vi "Create.vi"(7 "Direction":T1, 8 "error in (no error)":errorcluster, 9 "Custom Config Data":u8[](array[numeric]), 10 "Name":string, 11 "CIF_NIChn_FIFO_DAQ in":refnum<class "CIF_NIChn_DAQ_Base.lvclass">) -> (0 "error out":errorcluster, 3 "CIF_NIChn_FIFO_DAQ out":refnum<class "CIF_NIChn_DAQ_Base.lvclass">)   [LabVIEW 2021, in "CIF_NIChn_DAQ_Base.lvclass"]
uses:
  CIF_NIChn_DAQ_Base.lvclass
  D:/dev/Packages/CIF_Channels_Core/src/CIFChannels/CIFChannels.lvclass
  D:/dev/Packages/CIF_Channels_Core/src/CIF_NIChn/NIChn/CIF_NIChn.lvclass
  D:/dev/Packages/CIF_Channels_Core/src/CIF_NIChn/FIFO_U8/CIF_NIChn_Fifo_U8.lvclass
  CIFChannels/Typedef/Direction.ctl
  <vilib>/CIF Foundation/CIF Utilities/Statistics/I64/Stats_I64_CIF_U.lvclass/Stats_I64_CIF_U.ctl
  CIFChannels/Typedef/Disconnect Behavior.ctl
  CIFChannels/CIFChannels.lvclass/CIFChannels.ctl
  Typedef/Datatype Waveform Channel.ctl
  CIFChannels/Typedef/Channel State.ctl
  CIF_NIChn_DAQ_Base.lvclass/CIF_NIChn_DAQ_Base.ctl
  NIChn/CIF_NIChn.lvclass/CIF_NIChn.ctl
  FIFO_U8/CIF_NIChn_Fifo_U8.lvclass/CIF_NIChn_Fifo_U8.ctl
  5b466fd0-ea5b-47e1-b1f3-5756b43c2cf4.vi
  92f6609d-ad7c-4ed0-9d81-d11473a8d94d.vi
  CIFChannels/Accessors/Write Channel State.vi
  NIChn/Accessors/Write CIF Channel.vi
  CIFChannels/Accessors/Write Channel Benchmark.vi
  CIFChannels/Accessors/Write Flatten Benchmark.vi
  FIFO_U8/Accessors/Write Payload.vi
  CIFChannels/SubVIs/Get Type from Class.vi
  ChannelCommon/Utilities/Unflatten FIFO Config.vi
  CIFChannels/Utilities/Apply Flags.vi
  CIFChannels/Accessors/Write Type.vi
  CIFChannels/Accessors/Write Channel Class.vi
  CIFChannels/Accessors/Write Direction.vi
  CIFChannels/Accessors/Write Tag Disconnect Behavior.vi
  CIFChannels/Accessors/Write Name.vi
  CIFChannels/Accessors/Write Custom Config Data.vi
  <vilib>/CIF Foundation/NI Channels/SubVIs/Add Error.vi
  5b466fd0-ea5b-47e1-b1f3-5756b43c2cf4.vi/c28b0ead-42ad-4072-80a2-aca7f2bd7ce3.vi
  <vilib>/CIF Foundation/NI Channels/SubVIs/CIFServices Fill In Error Info Ex.vi
  <vilib>/CIF Foundation/NI Channels/SubVIs/Get dll Path.vi
  5b466fd0-ea5b-47e1-b1f3-5756b43c2cf4.vi/259f1102-a6f3-45ef-83a9-e8a266e5a7b9.vi
  92f6609d-ad7c-4ed0-9d81-d11473a8d94d.vi/c28b0ead-42ad-4072-80a2-aca7f2bd7ce3.vi
  <vilib>/CIF Foundation/CIF Utilities/DataTypes/Unflatten U64.vi
  ChannelCommon/Utilities/Expand FIFO Flags.vi
  <vilib>/CIF Foundation/CIF Utilities/Errors/Append Error Location.vi
  <vilib>/Utility/LVClass/Get LV Class Name.vi
  <vilib>/CIF Foundation/CIF Utilities/Statistics/I64/Stats_I64_CIF_U.lvclass
  CIFChannels/CIFChannels.lvclass
  ChannelCommon/ChannelCommon.lvlib
  ChannelCommon/typedef/Channel Pattern.ctl
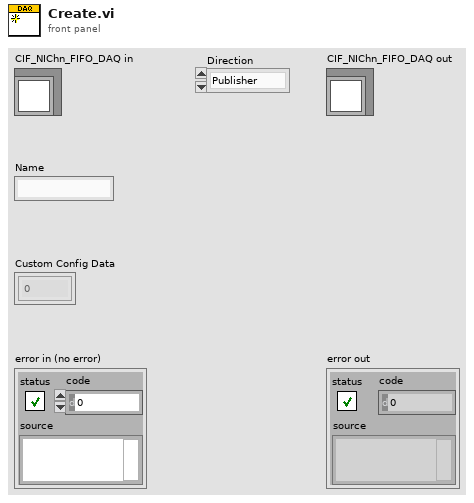
[diagram p1: front panel]
types:
  T1 = typedef "CIFChannels.lvclass/Direction.ctl" = enum16{"Publisher", "Subscriber"}
  T2 = typedef "ChannelCommon.lvlib/Channel Pattern.ctl" = enum16{"Unknown", "Tag", "FIFO", "MultiFIFO"}
  T3 = typedef "CIFChannels.lvclass/Disconnect Behavior.ctl" = enum16{"Default value", "Last value", "Error with default"}
  T4 = typedef "CIF_NIChn_DAQ_Base.lvclass/Datatype Waveform Channel.ctl" = cluster{"measurement":dbl[], "dT":dbl, "Timestamp":i64, "Read Lock":bool}
  T5 = typedef "CIFChannels.lvclass/Channel State.ctl" = enum16{"Creating", "Disconnected", "Connecting", "Connected", "Destroyed"}
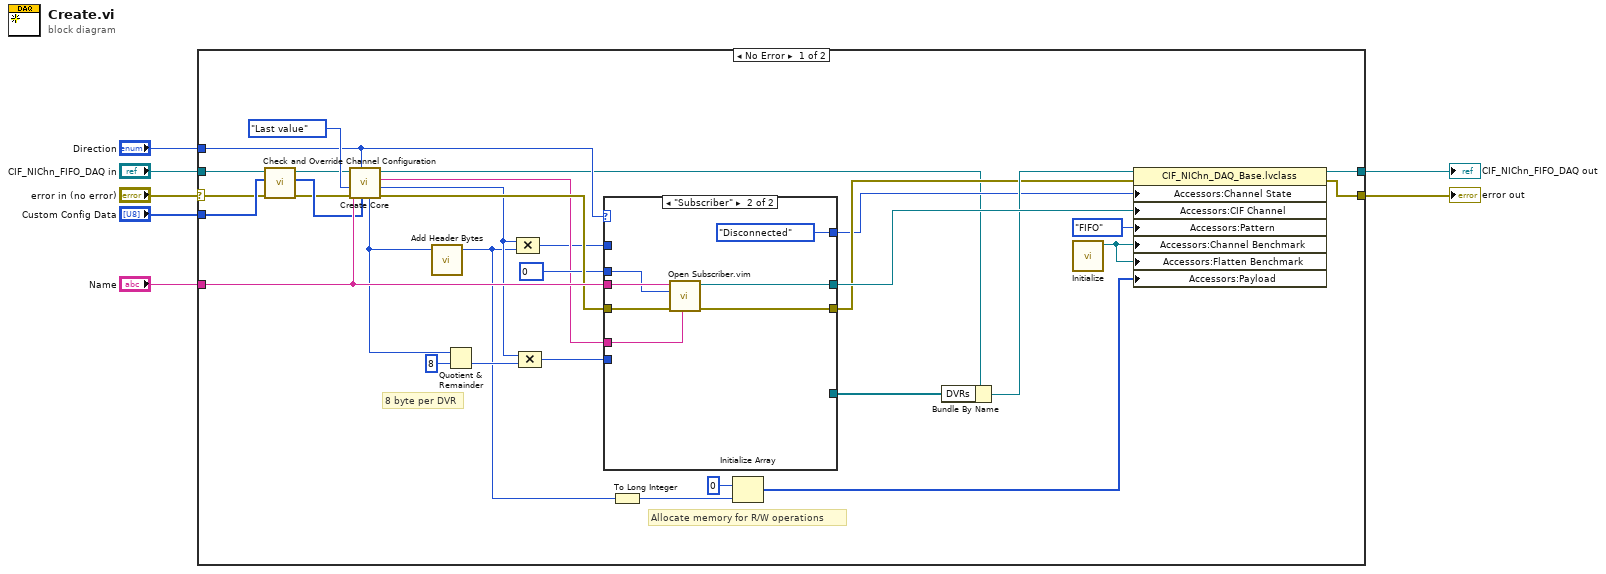
[diagram p0: block diagram]
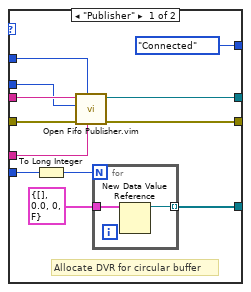
[diagram p2: hidden frame]
diagram:
  n1 = case shown="No Error" "error in (no error)" {
    selector: "error in (no error)" -> [w13 w62]
    tunnel: [w38 w62] -> w6
    tunnel: [w32 w61] -> w1
    tunnel: "CIF_NIChn_FIFO_DAQ in" -> [w16 w61]
    tunnel: "Name" -> [w37 _]
    tunnel: "Direction" -> [w31 _]
    tunnel: "Custom Config Data" -> [w15 _]
    frame No Error {
      # "8 byte per DVR"
      # "Allocate memory for R/W operations"
      n2 = call-dynamic "Check and Override Channel Configuration.vi"("error in (no error)"=w13, "Custom Config Data in"=w15, "CIF_NIChn_FIFO_DAQ in"=w16) -> ("error out"=w12:errorcluster, "Custom Config Data out"=w14:u8[], "CIF_NIChn_FIFO_DAQ out"=w11:refnum<class "CIF_NIChn_DAQ_Base.lvclass">)  [unwired: 6 in]
      n3 = call "Create Core.vi"("Custom Config Data"=w14, "Direction"=w31, "error in (no error)"=w12, "Disconnect Behavior"=Disconnect_Behavior."Last value", "Name"=w37, "CIFChannels in"=w11) -> ("error out"=w36:errorcluster, "Messages"=w19:u64, "Channel Type"=w28:string, "CIFChannels out"=w10:refnum<class "CIF_NIChn_DAQ_Base.lvclass">, "Bytes/Msg"=w18:u64)  [unwired: 1 in]
      n4 = call "Add Header Bytes.vi"("Bytes/Msg"=w18) -> ("Bytes/Msg with header"=w17:u64)  [unwired: 3 in]
      n5 = Quotient & Remainder(x=w18, y=u64 8) -> (floor(x/y)=w22:u64)  [unwired: 1 out]
      n6 = Compound Arithmetic op=MULTIPLY(w19, w17) -> (w26:u64)
      n7 = Compound Arithmetic op=MULTIPLY(w19, w22) -> (w21:u64)
      n8 = case shown="\"Subscriber\"" w31 {
        tunnel: w37 -> [w51 w59]
        tunnel: w36 -> [w50 w58]
        tunnel: [w46 w54] -> w35
        tunnel: [w47 w55] -> w33
        tunnel: w28 -> [w49 w57]
        tunnel: [Channel_State."Connected" ("Channel State") Channel_State."Disconnected" ("Channel State")] -> w30
        tunnel: u8 0 -> [w45 w56]
        tunnel: w26 -> [w44 _]
        tunnel: w21 -> [w41 _]
        tunnel: [w43 _] -> w25
        frame "Publisher" {
          # "Allocate DVR for circular buffer"
          n9 = To Long Integer(number=w41) -> (32bit integer=w40:i32)
          n10 = call "Open Fifo Publisher.vim"("Channel Type Description"=w49, "depth"=w44, "error in"=w50, "Input Type"=w45, "Channel Name"=w51) -> ("error out"=w47:errorcluster, "CIF Channel"=w46:refnum<k21>)  [unwired: 5 in]
          n11 = for {
            N: w40 -> [_]
            tunnel: T4 {"measurement"=[], "dT"=0.0, "Timestamp"=0, "Read Lock"=FALSE} ("Waveform Datatype") -> [w53]
            tunnel: [w52] -> w43 mode=indexing
            n12 = New Data Value Reference(data value=w53) -> (data value reference=w52:refnum<data-value>)  [unwired: 1 in, 1 out]
          }
        }
        frame "Subscriber" {
          n13 = call "Open Subscriber.vim"("Channel Type Description"=w57, "error in"=w58, "Input Type"=w56, "Channel Name"=w59) -> ("error out"=w55:errorcluster, "CIF Channel"=w54:refnum<k21>)  [unwired: 6 in]
        }
      }
      n14 = To Long Integer(number=w17) -> (32bit integer=w20:i32)
      n15 = Initialize Array(u8 0 ("Numeric"), w20) -> (w9:u8[])
      n16 = Bundle By Name(cluster=w10, "DVRs"=w25) -> (w34:refnum<class "CIF_NIChn_DAQ_Base.lvclass">)
      n17 = call <vilib>:"Initialize.vi"() -> ("Stats_I64_CIF_U out"=w24:refnum<class "Stats_I64_CIF_U.lvclass">)  [unwired: 10 in, 1 out]
      n18 = property class="CIF_NIChn_DAQ_Base.lvclass"(reference=w34, error in=w33, "Accessors:Channel State"=w30, "Accessors:CIF Channel"=w35, "Accessors:Pattern"=Channel_Pattern."FIFO" ("Pattern"), "Accessors:Channel Benchmark"=w24, "Accessors:Flatten Benchmark"=w24, "Accessors:Payload"=w9) -> (reference out=w32:refnum<class "CIF_NIChn_DAQ_Base.lvclass">, error out=w38:errorcluster)
    }
    frame Error {
    }
  }
  "CIF_NIChn_FIFO_DAQ out" <- w1
  "error out" <- w6
